vi "Read Self Attributes.vi"(7 "Actor in":refnum<class "Actor.lvclass">) -> (2 "Self Attributes":refnum<data-value>)   [LabVIEW 2020, in "jettl.lvlib" / "Actor Specific.lvlib"]
uses:
  Actor Specific.lvlib
  Actor/Actor.lvclass
  Transport/Transport.lvclass
  Actor Attributes.ctl
  jettl.lvlib
  Msg/Msg.lvclass
  Msgs.ctl
  Msg Names.ctl
  Unified Layer.ctl
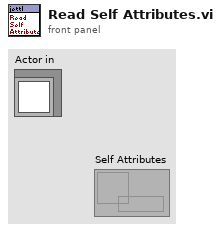
[diagram p1: front panel]
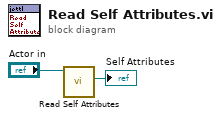
[diagram p0: block diagram]
diagram:
  n1 = call-dynamic "Read Self Attributes.vi"("Actor in"="Actor in") -> ("Self Attributes"=→"Self Attributes":refnum<data-value>)  [unwired: 10 in]
